vi "Tip tune ZaberAndSR865.vi"(0 "Z axis":T3={"Serial port handle"="", "Axis"="", "Controller #"=0, "Min position"=0.0, "Max position"=0.0, "Min velocity"=0.0, "Max velocity"=0.0, "Firmware"="", "Device ID"=0, "Variable event"=refnum, "Variable ref"=refnum, "Resolution, usteps/step"=0, "Serial port semaphore"=refnum, "Joystick buttons"={"MinDir"=1, "MaxDir"=2, "MedSpeed"=5, "HighSpeed"=6}} {"Joystick buttons"."HighSpeed" min=1 max=25 step=1; "Joystick buttons"."MedSpeed" min=1 max=25 step=1; "Joystick buttons"."MaxDir" min=1 max=25 step=1; "Joystick buttons"."MinDir" min=1 max=25 step=1}, 1 "SR865":T1, 2 "Stop event":refnum<user-event>, 5 "error in":errorcluster) -> (19 "error out":errorcluster)   [LabVIEW 2018]
uses:
  Zaber library/Zaber.ctl
  GenericDataEvent/GenericEvent.ctl
  Zaber library/ZaberVariables.ctl
  SR865/SR865.ctl
  SR865/OutSineReference.ctl
  SR865/OutSineSource.ctl
  SR865/DataChannel.ctl
  <vilib>/Analysis/6fits.llb/Curve Fitting Criteria.ctl
  <vilib>/Analysis/NI_AAL_SigProc.lvlib
  <vilib>/Analysis/NI_AALBase.lvlib
  <vilib>/Analysis/NI_AALPro.lvlib
panel:
  in  "btnReadSignal":bool
  out "Signal":dbl=100000.0 caption="Signal, mV"
  in  "BtnZ-":bool
  in  "BtnZ+":bool
  in  "ZStep":dbl=0.005 caption="Z step, mm" min=0.0 max=25.0 step=0.01 format="%#.4f"
  in  "btnStartPosScanning":bool caption="stop"
  in  "btnCalculateSlope":bool
  in  "btnCalculateSurfaceLevel":bool
  in  "btnCalculateAirLevel":bool
  out "FrequencyStepRb":dbl=100000.0 caption="Frequency"
  out "PhaseRb":dbl=100000.0 caption="Frequency"
  out "AmplitudeRb":dbl=100000.0 caption="Frequency"
  out "DCOffsetRb":dbl=100000.0 caption="DC offset, V"
  out "SlopeError":dbl=8.6 caption="Slope error, V/mm" min=0.0 max=25.0 step=0.01 format="%#.4f"
  out "SurfaceError":dbl=8.6 caption="Surface error, V" min=0.0 max=25.0 step=0.01 format="%#.4f"
  out "AirError":dbl=8.6 caption="Air error, V" min=0.0 max=25.0 step=0.01 format="%#.4f"
  out "Slope":dbl=8.6 caption="Slope, mm/V" min=0.0 max=25.0 step=0.01 format="%#.4f"
  out "SurfaceLevel":dbl=8.6 caption="Surface level, V" min=0.0 max=25.0 step=0.01 format="%#.4f"
  out "AirLevel":dbl=8.6 caption="Air level, V" min=0.0 max=25.0 step=0.01 format="%#.4f"
  out "CurrentStep":i32=61 caption="Z steps"
  out "PltScanningPosition":cluster{dbl[], dbl[]}[](graph) caption="Position scanning"
  out "ZStep":dbl=0.0016666666666666607 caption="Z step, mm" min=0.0 max=25.0 format="%#.4f"
  in  "Frequency":dbl=97044.98 caption="Frequency, Hz" format="%.2p"
  in  "BtnSetZEndPosition":bool
  in  "BtnSetZStartPosition":bool
  in  "ZPoints":i32=61 caption="Z points"
  out "ZEndPosition":dbl=8.6 caption="Z end, mm" min=0.0 max=25.0 format="%#.4f"
  out "ZStartPosition":dbl=8.5 caption="Z start, mm" min=0.0 max=25.0 format="%#.4f"
  out "ZPositionRb":dbl=8.6 caption="Z position" min=0.0 max=25.0 step=0.01 format="%#.4f"
  in  "ZPosition":dbl=8.5 caption="Z position, mm" min=0.0 max=25.0 step=0.01 format="%#.4f"
  out "TblBestFrequencyies":string[][](table)=[["97044.98", "2.85"], ["82864.39", "1.68"], ["21141.21", "1.26"], ["93904.03", "0.82"], ["15778.11", "0.52"]] caption="Best frequencies, Hz"
  in  "TipPlace":u16(ring)=1 caption="Tip place" items=["Air", "Surface"]
  in  "SettingTime":u32=1000 caption="Setting time, ms"
  out "FrequencyRb":dbl=100000.0 caption="Frequency"
  out "CurrentPoint":i32=90
  out "PltScanningFrequence":cluster{dbl[], dbl[]}[](graph)=[{[10000.0, 11000.0, 12000.0, 13000.0, 14000.0, 15000.0, 16000.0, 17000.0, 18000.0, 19000.0, 20000.0, 21000.0, 22000.0, 23000.0, 24000.0, 25000.0, 26000.0, 27000.0, 28000.0, 29000.0, 30000.0, 31000.0, 32000.0, 33000.0, 34000.0, 35000.0, 36000.0, 37000.0, 38000.0, 39000.0, 40000.0, 41000.0, 42000.0, 43000.0, 44000.0, 45000.0, 46000.0, 47000.0, 48000.0, 49000.0, 50000.0, 51000.0, 52000.0, 53000.0, 54000.0, 55000.0, 56000.0, 57000.0, 58000.0, 59000.0, 60000.0, 61000.0, 62000.0, 63000.0, 64000.0, 65000.0, 66000.0, 67000.0, 68000.0, 69000.0, 70000.0, 71000.0, 72000.0, 73000.0, 74000.0, 75000.0, 76000.0, 77000.0, 78000.0, 79000.0, 80000.0, 81000.0, 82000.0, 83000.0, 84000.0, 85000.0, 86000.0, 87000.0, 88000.0, 89000.0, 90000.0, 91000.0, 92000.0, 93000.0, 94000.0, 95000.0, 96000.0, 97000.0, 98000.0, 99000.0, 100000.0], [3.5655190000512516, 3.4374305005139005, 3.4273711461139715, 3.4850248112142093, 3.5761130550998383, 3.556590231281875, 3.5082421792498932, 3.012145327734691, 3.60479334690102, 3.6237170567298436, 3.5213679819034964, 4.863866373270507, 4.004233765623082, 3.958662171251218, 3.638372868429504, 3.6863311988676024, 3.6407628928169347, 3.597268956374069, 3.472475578654757, 3.4138362740831423, 4.023460288827825, 3.8711427099095466, 3.8072787456116726, 3.773067870768127, 3.802872335674139, 3.843425482975206, 3.8131604010931146, 3.710485915669144, 3.68892415072003, 3.7175819077370553, 3.6497045488279003, 3.698426272759254, 3.738228894609222, 3.7572105957332433, 3.841541162636644, 3.552982648310411, 3.6359506328697484, 3.7367182179969376, 3.817937233155462, 3.940743403433729, 4.337961900873752, 3.232249392203631, 3.031809835447508, 3.1009883283630275, 3.1785447948663723, 2.9738534939166783, 3.794967857187948, 3.786370846678634, 3.691365712894553, 3.655859990170908, 3.6562916119155986, 3.5957679438322634, 3.593065477052433, 3.5925726553448727, 3.5922634338806207, 3.590250273321926, 3.597758557035468, 3.5946888897478324, 3.606027010467748, 3.573291409437125, 3.5650938203985896, 3.532467740941366, 3.385655269781037, 3.651862657728945, 3.6418741576807374, 3.5802843235408948, 3.611222575631784, 3.5164236610651676, 4.632535226763082, 3.2424697969441687, 3.272032610844888, 3.3549199729897623, 3.7972193768166784, 5.452081044437504, 2.748058067103696, 2.9130046647694234, 2.9576226283303546, 3.0336329490386387, 3.0499346821806705, 2.9810010016675736, 2.8330872460617447, 2.3801761264752517, 1.3887019949256822, 6.48560906859755, 5.721885978735551, 3.7523307011355125, 2.996072291328326, 5.390088024437564, 5.438011320322094, 4.595058047439225, 4.5440910275334865]}, {[10000.0, 11000.0, 12000.0, 13000.0, 14000.0, 15000.0, 16000.0, 17000.0, 18000.0, 19000.0, 20000.0, 21000.0, 22000.0, 23000.0, 24000.0, 25000.0, 26000.0, 27000.0, 28000.0, 29000.0, 30000.0, 31000.0, 32000.0, 33000.0, 34000.0, 35000.0, 36000.0, 37000.0, 38000.0, 39000.0, 40000.0, 41000.0, 42000.0, 43000.0, 44000.0, 45000.0, 46000.0, 47000.0, 48000.0, 49000.0, 50000.0, 51000.0, 52000.0, 53000.0, 54000.0, 55000.0, 56000.0, 57000.0, 58000.0, 59000.0, 60000.0, 61000.0, 62000.0, 63000.0, 64000.0, 65000.0, 66000.0, 67000.0, 68000.0, 69000.0, 70000.0, 71000.0, 72000.0, 73000.0, 74000.0, 75000.0, 76000.0, 77000.0, 78000.0, 79000.0, 80000.0, 81000.0, 82000.0, 83000.0, 84000.0, 85000.0, 86000.0, 87000.0, 88000.0, 89000.0, 90000.0, 91000.0, 92000.0, 93000.0, 94000.0, 95000.0, 96000.0, 97000.0, 98000.0, 99000.0, 100000.0], [3.6968028657407785, 3.397109339181018, 3.567193952093816, 3.4622519508906793, 3.5945342790368535, 3.5386940424582525, 3.029648511216874, 3.7294031949868516, 3.854496267967221, 3.66608362794549, 3.6337442084525384, 3.622335223134029, 3.520269601833684, 3.625449985669437, 3.5996783070122036, 3.596367060420739, 3.6706800775467205, 3.6178547324397927, 3.494530145248237, 3.4783507835572123, 3.9798696462301795, 3.909521653058709, 3.84636309009401, 3.8283541416529783, 3.8855956102501024, 3.948232372330415, 3.8955390259265563, 3.7044271046719377, 3.6476140823855085, 3.685313344462496, 3.639751480735465, 3.690521795627914, 3.727960158953497, 3.75535848669949, 3.8145229094921054, 3.5935582988975963, 3.6440902453414807, 3.730672290482194, 3.7940627371494946, 3.884890197869988, 4.123519414820418, 5.233578709141258, 2.8898807738384256, 2.709737263826195, 3.650699858167375, 3.6058691787236263, 3.5725795559217843, 3.585563635600408, 3.5978873993164835, 3.6012115301523817, 3.545358407800998, 3.557833559064785, 3.5697611313701043, 3.5699866053317777, 3.5644109564113067, 3.568540350922504, 3.570524521787714, 3.5653418417511418, 3.5472878205078633, 3.566549737959607, 3.5284381997956884, 3.443283156254747, 3.726391503493266, 3.6588555739683373, 3.5487920538102036, 3.744426212291304, 3.774333747133092, 3.7278280955270975, 4.291694487008893, 3.381445353898666, 3.4274420088262834, 3.5326255726860984, 3.8970271568359123, 3.8148611207822927, 4.140697353288415, 3.4812175242568655, 3.7482206201906454, 2.959581027358073, 2.755453572987086, 2.842289778548217, 2.8230407994627473, 2.5397852639697267, 1.7720535165304037, 6.311279502338936, 4.911483553972613, 3.8801745664846505, 3.1735908186482717, 2.5479667164400683, 5.117117280660982, 5.956381695510879, 6.236143926446963]}, {[10000.0, 11000.0, 12000.0, 13000.0, 14000.0, 15000.0, 16000.0, 17000.0, 18000.0, 19000.0, 20000.0, 21000.0, 22000.0, 23000.0, 24000.0, 25000.0, 26000.0, 27000.0, 28000.0, 29000.0, 30000.0, 31000.0, 32000.0, 33000.0, 34000.0, 35000.0, 36000.0, 37000.0, 38000.0, 39000.0, 40000.0, 41000.0, 42000.0, 43000.0, 44000.0, 45000.0, 46000.0, 47000.0, 48000.0, 49000.0, 50000.0, 51000.0, 52000.0, 53000.0, 54000.0, 55000.0, 56000.0, 57000.0, 58000.0, 59000.0, 60000.0, 61000.0, 62000.0, 63000.0, 64000.0, 65000.0, 66000.0, 67000.0, 68000.0, 69000.0, 70000.0, 71000.0, 72000.0, 73000.0, 74000.0, 75000.0, 76000.0, 77000.0, 78000.0, 79000.0, 80000.0, 81000.0, 82000.0, 83000.0, 84000.0, 85000.0, 86000.0, 87000.0, 88000.0, 89000.0, 90000.0, 91000.0, 92000.0, 93000.0, 94000.0, 95000.0, 96000.0, 97000.0, 98000.0, 99000.0, 100000.0], [-0.131283865689527, 0.04032116133288266, -0.1398228059798443, 0.022772860323529986, -0.018421223937015174, 0.017896188823622428, 0.47859366803301917, -0.7172578672521608, -0.24970292106620118, -0.04236657121564624, -0.112376226549042, 1.2415311501364776, 0.4839641637893983, 0.3332121855817811, 0.03869456141730021, 0.08996413844686346, -0.029917184729785884, -0.02058577606572376, -0.02205456659347993, -0.06451450947407, 0.043590642597645335, -0.03837894314916257, -0.03908434448233722, -0.05528627088485116, -0.0827232745759634, -0.10480688935520899, -0.08237862483344172, 0.0060588109972061766, 0.04131006833452133, 0.03226856327455918, 0.009953068092435124, 0.007904477131339682, 0.01026873565572517, 0.0018521090337535462, 0.02701825314453865, -0.04057565058718504, -0.008139612471732338, 0.006045927514743532, 0.023874496005967583, 0.05585320556374107, 0.2144424860533345, -2.0013293169376274, 0.14192906160908247, 0.39125106453683234, -0.47215506330100254, -0.632015684806948, 0.2223883012661636, 0.2008072110782262, 0.09347831357806946, 0.05464846001852619, 0.1109332041146005, 0.037934384767478235, 0.02330434568232853, 0.022586050013094994, 0.027852477469314074, 0.021709922399422155, 0.02723403524775403, 0.029347047996690634, 0.05873918995988481, 0.006741671477517919, 0.03665562060290117, 0.08918458468661905, -0.3407362337122293, -0.006992916239392244, 0.09308210387053384, -0.16414188875040914, -0.16311117150130805, -0.2114044344619299, 0.3408407397541886, -0.13897555695449748, -0.15540939798139553, -0.17770559969633615, -0.09980778001923385, 1.6372199236552114, -1.392639286184719, -0.568212859487442, -0.7905979918602908, 0.07405192168056551, 0.2944811091935846, 0.13871122311935657, 0.010046446598997338, -0.15960913749447503, -0.3833515216047214, 0.1743295662586144, 0.8104024247629376, -0.12784386534913805, -0.17751852731994555, 2.842121307997496, 0.32089403966111174, -1.3613236480716537, -1.6920528989134764]}] caption="Frequence scanning"
  in  "btnStartFreqScanning":bool caption="stop"
  out "FrequencyPoints":i32=91 caption="Frequency points"
  in  "FrequencyStep":dbl=1000.0 caption="Frequency step, Hz"
  in  "EndFrequency":dbl=100000.0 caption="End frequency, Hz" format="%.2p"
  in  "Phase":dbl format="%.3f"
  in  "StartFrequency":dbl=10000.0 caption="Start frequency, Hz" format="%.2p"
  in  "Amplitude":dbl=0.5 caption="Amplitude p-p, V" min=0.0 max=10.0 format="%.3f"
  # "RS865 parameters"
  # "Z stage parameters"
  # "Scanning parameters"
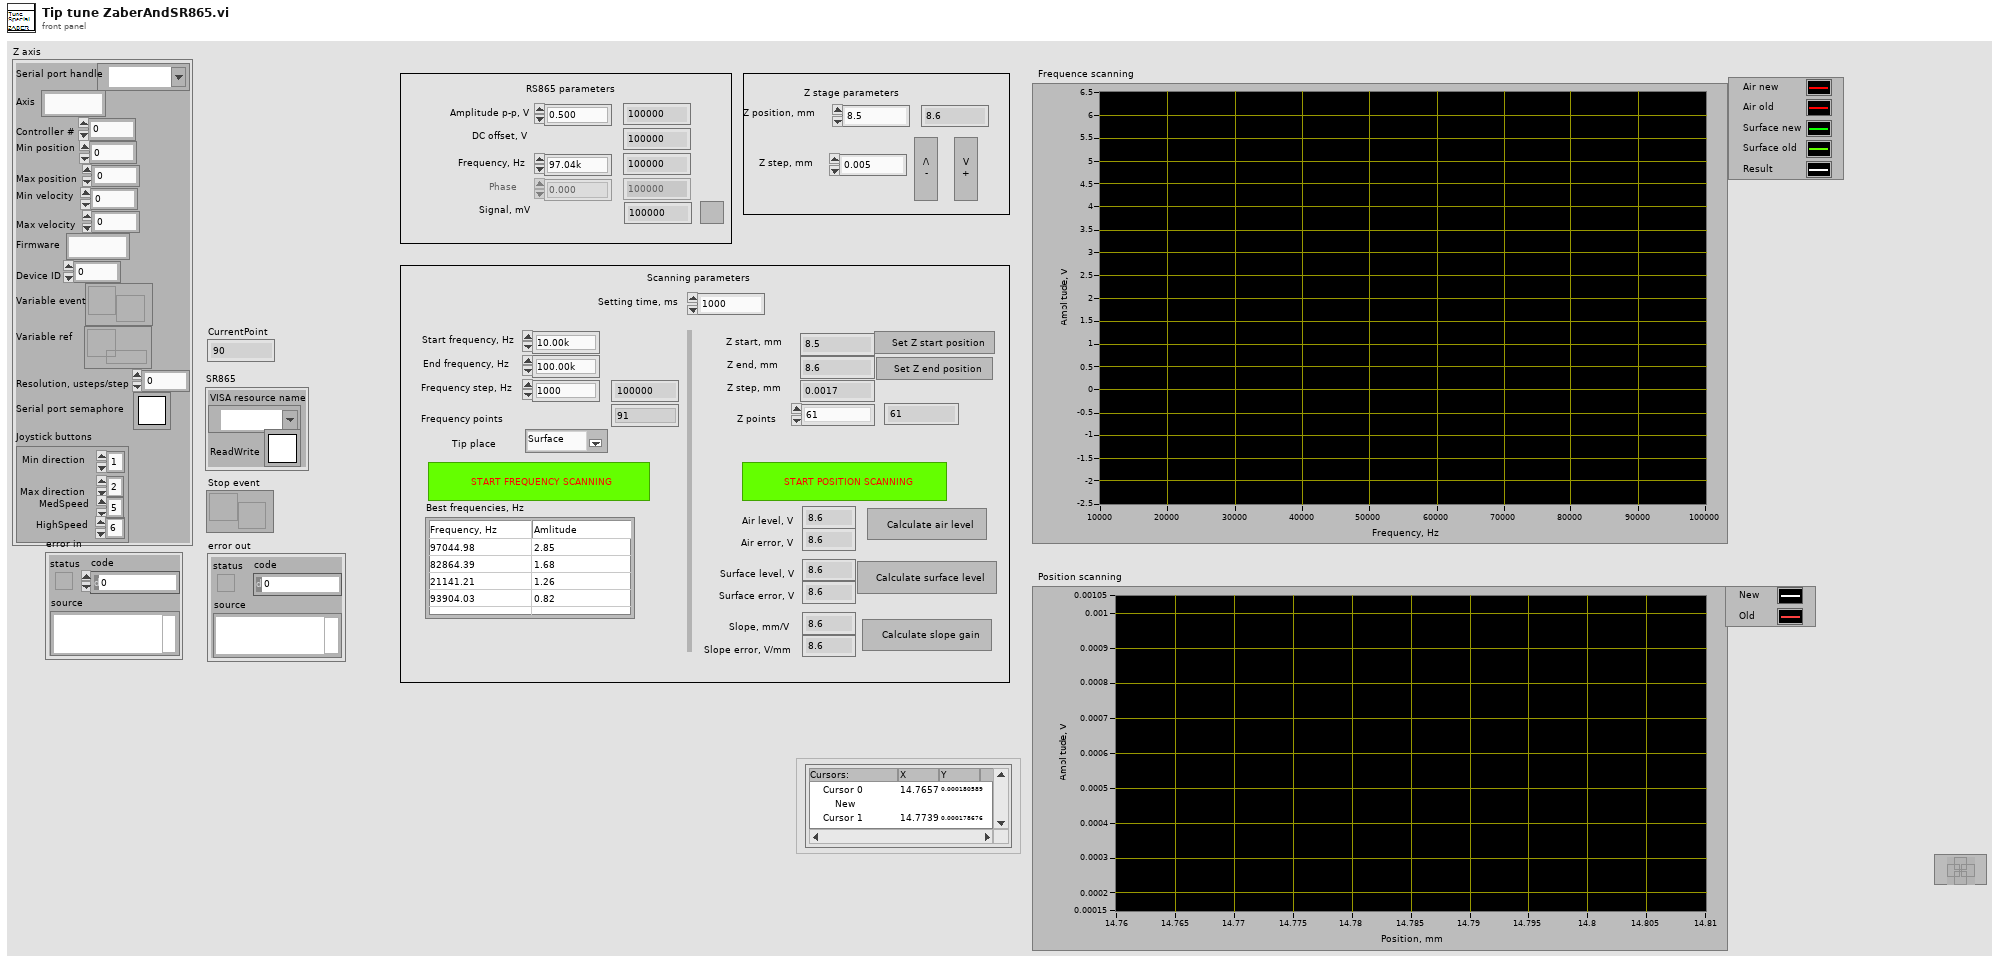
[diagram p1: front panel]
types:
  T1 = typedef "SR865.ctl" = cluster{"VISA resource name":refnum<visa-resource-name>, "ReadWrite":T2}
  T2 = typedef "Semaphore RefNum" = refnum<k1>
  T3 = typedef "Zaber.ctl" = cluster{"Serial port handle":refnum<visa-resource-name>, "Axis":string, "Controller #":u8, "Min position":dbl, "Max position":dbl, "Min velocity":dbl, "Max velocity":dbl, "Firmware":string, "Device ID":i32, "Variable event":T4, "Variable ref":refnum<data-value>, "Resolution, usteps/step":i32, "Serial port semaphore":T2, "Joystick buttons":cluster{"MinDir":i32, "MaxDir":i32, "MedSpeed":i32, "HighSpeed":i32}}
  T4 = typedef "GenericEvent.ctl" = refnum<user-event>
  T5 = typedef "DataChannel.ctl" = u16
  T6 = typedef "OutSineSource.ctl" = u16
  T7 = typedef "OutSineReference.ctl" = u16
  T8 = typedef "LVCursorListTypeDef.ctl" = cluster{"Name":string, "Color":u32, "Style":u8, "Point Style":u8, "Name Visible":bool, "Allow Drag":bool, "Cursor Mode":u32, "Plot":i32, "Index":i32, "Position":cluster{"X":dbl, "Y":dbl}, "X Scale":u32, "Y Scale":u32, "Watch Plots":i32[], "Watch All Plots":bool, "Plot Area":i32, "Label Offset":cluster{"X":dbl, "Y":dbl}}[]
  T9 = cluster{"Name":string, "Color":u32, "Style":u8, "Point Style":u8, "Name Visible":bool, "Allow Drag":bool, "Cursor Mode":u32, "Plot":i32, "Index":i32, "Position":cluster{"X":dbl, "Y":dbl}, "X Scale":u32, "Y Scale":u32, "Watch Plots":i32[], "Watch All Plots":bool, "Plot Area":i32, "Label Offset":cluster{"X":dbl, "Y":dbl}}
  T10 = typedef "NI_AALPro.lvlib/Curve Fitting Criteria.ctl" = u16
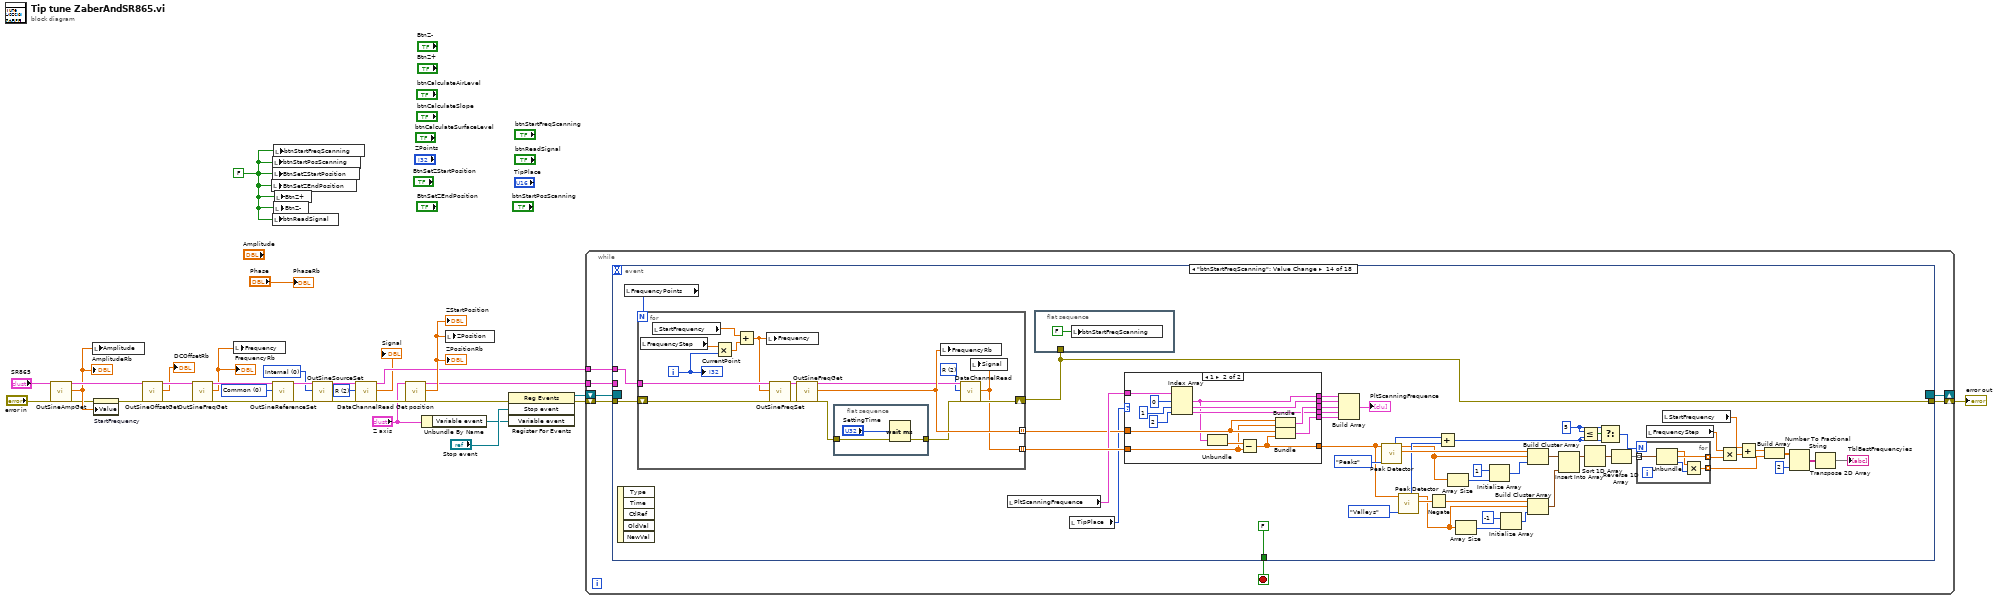
[diagram p0: block diagram]
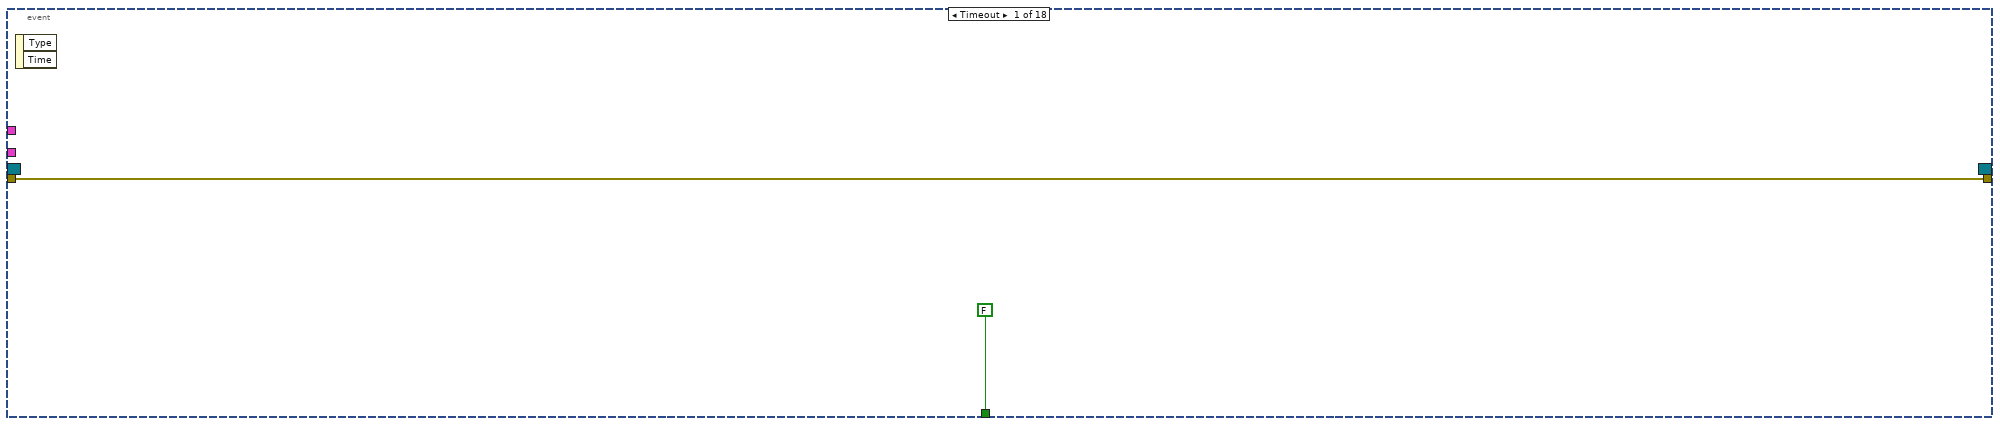
[diagram p2: hidden frame]
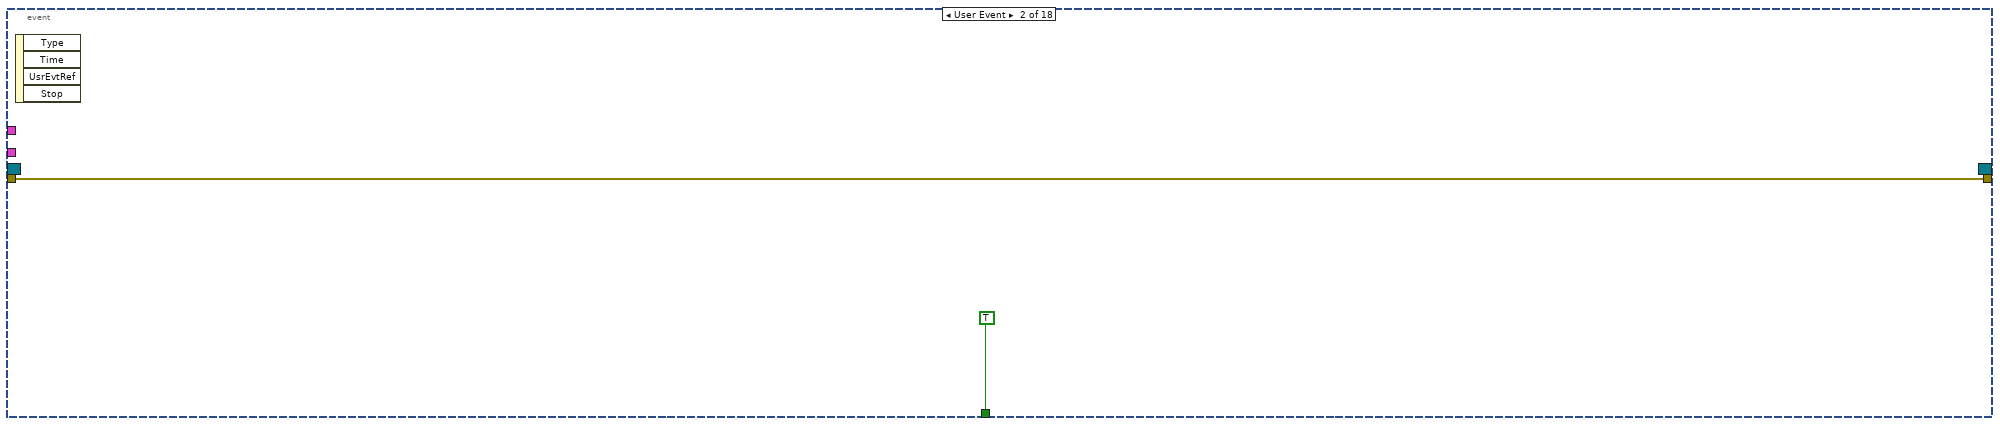
[diagram p3: hidden frame]
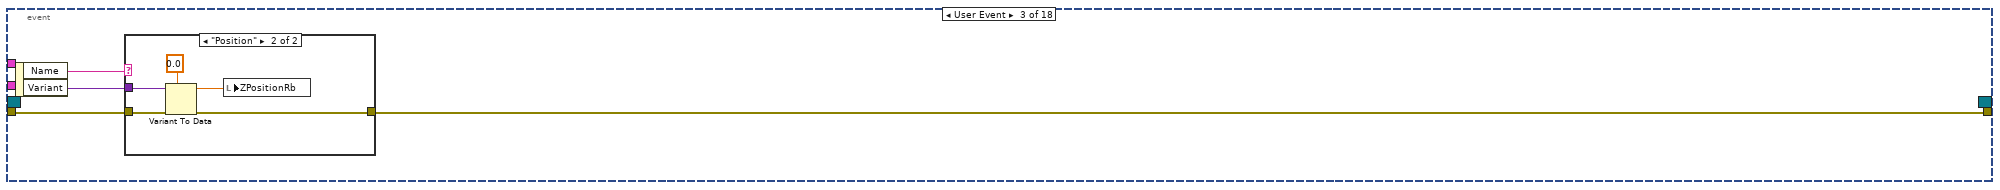
[diagram p4: hidden frame]
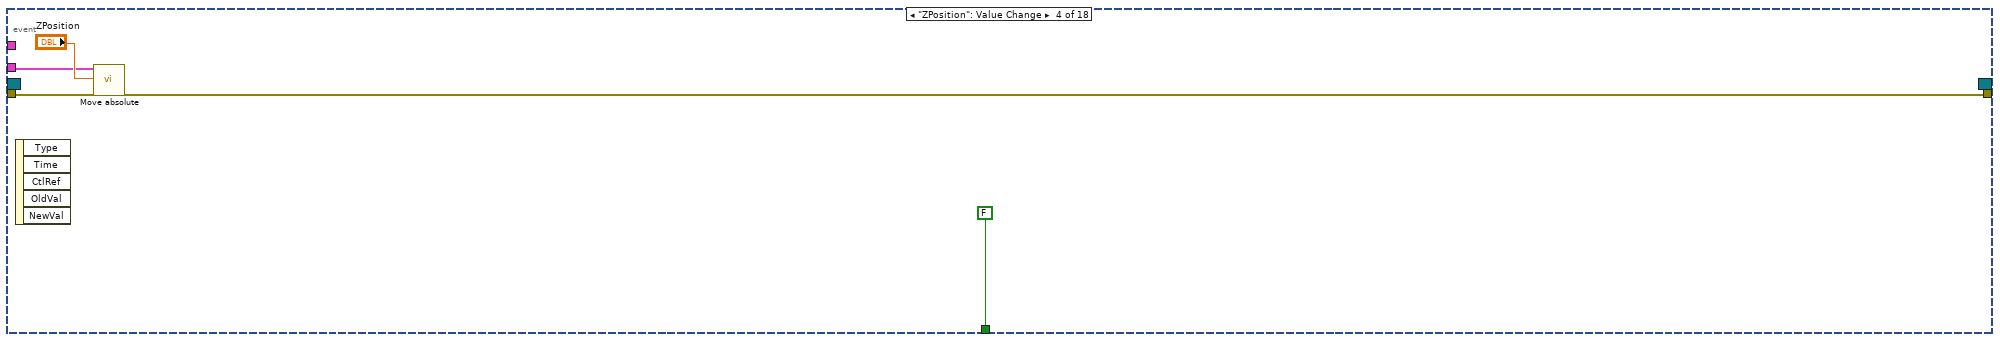
[diagram p6: hidden frame]
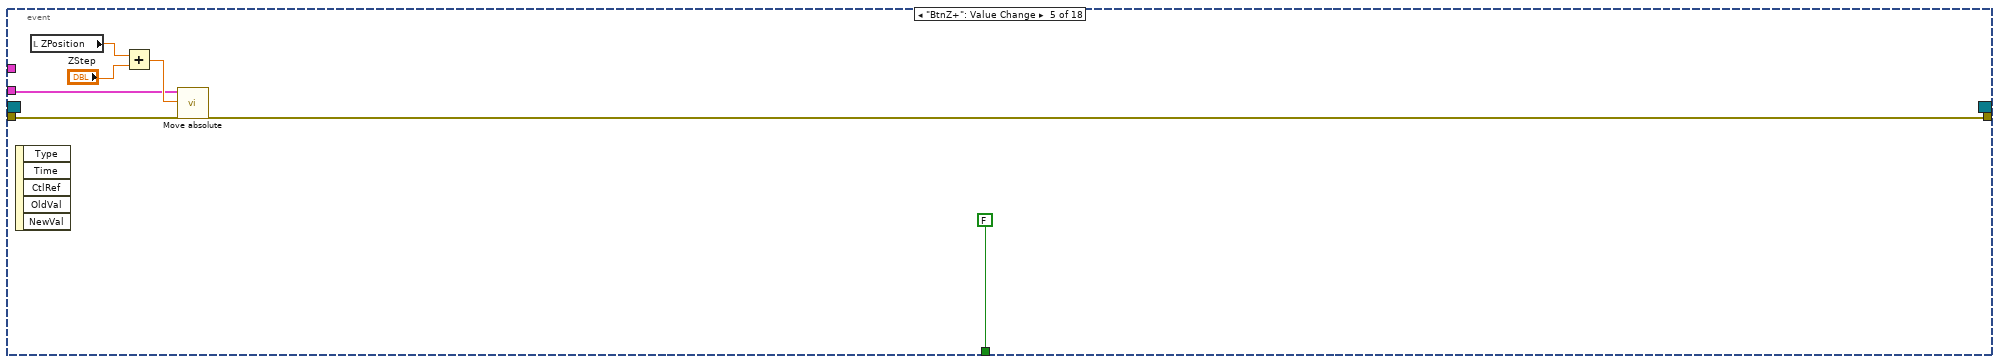
[diagram p7: hidden frame]
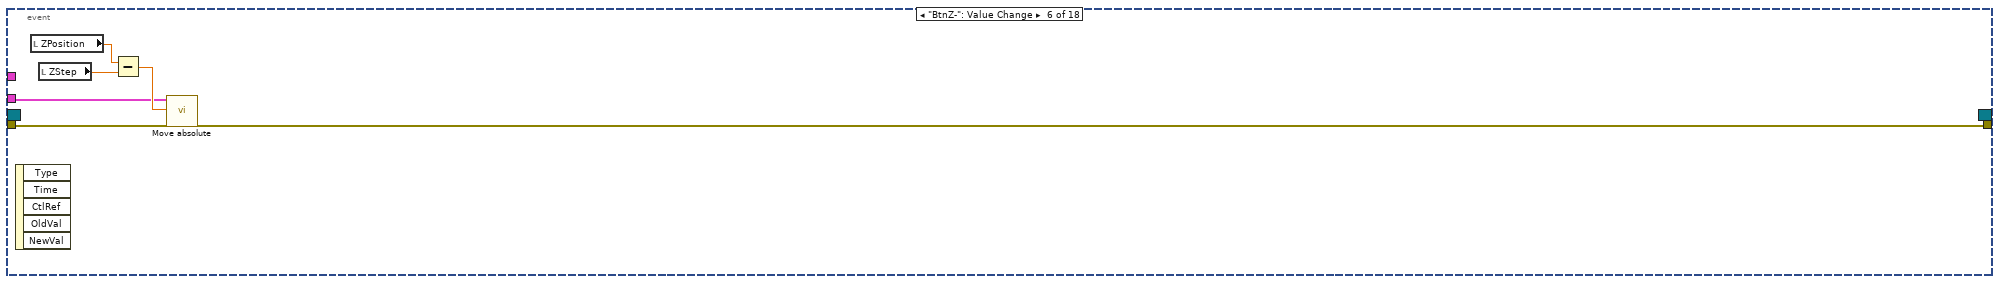
[diagram p8: hidden frame]
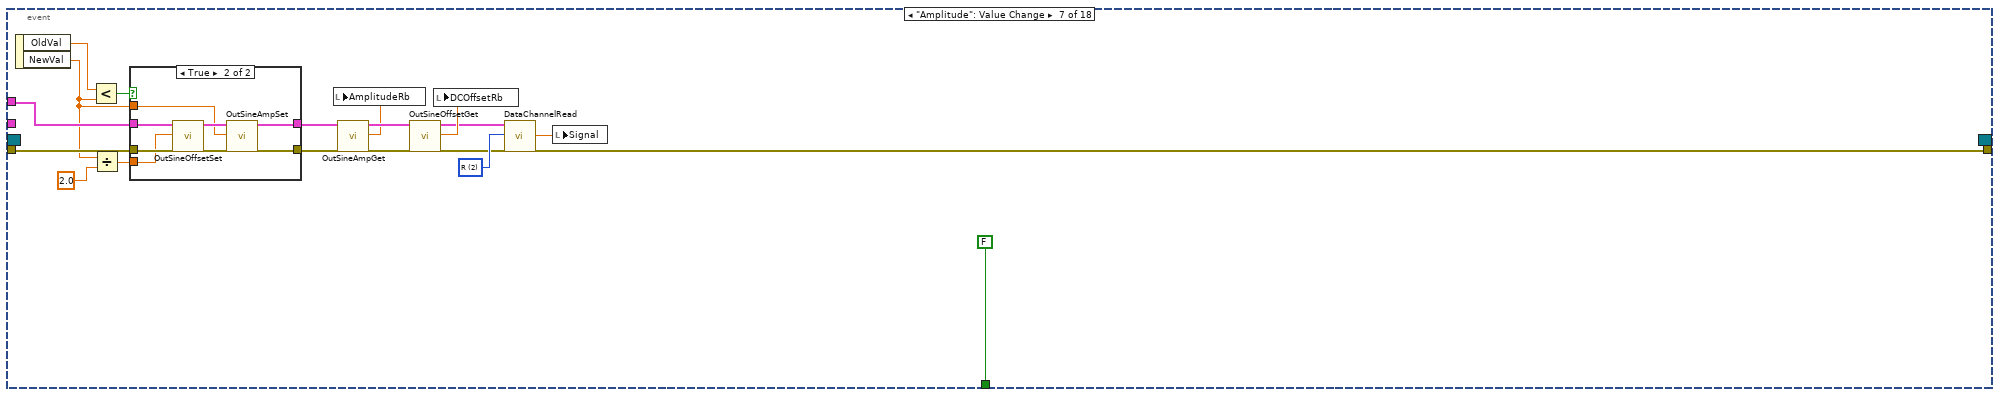
[diagram p9: hidden frame]
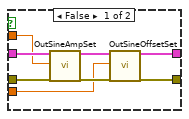
[diagram p10: hidden frame]
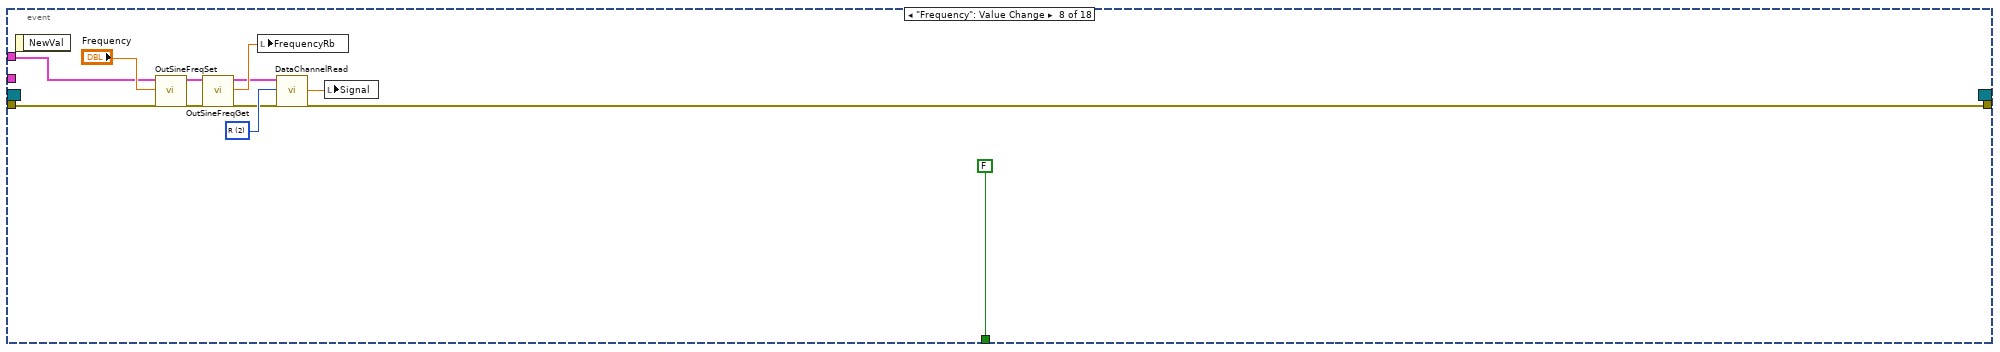
[diagram p11: hidden frame]
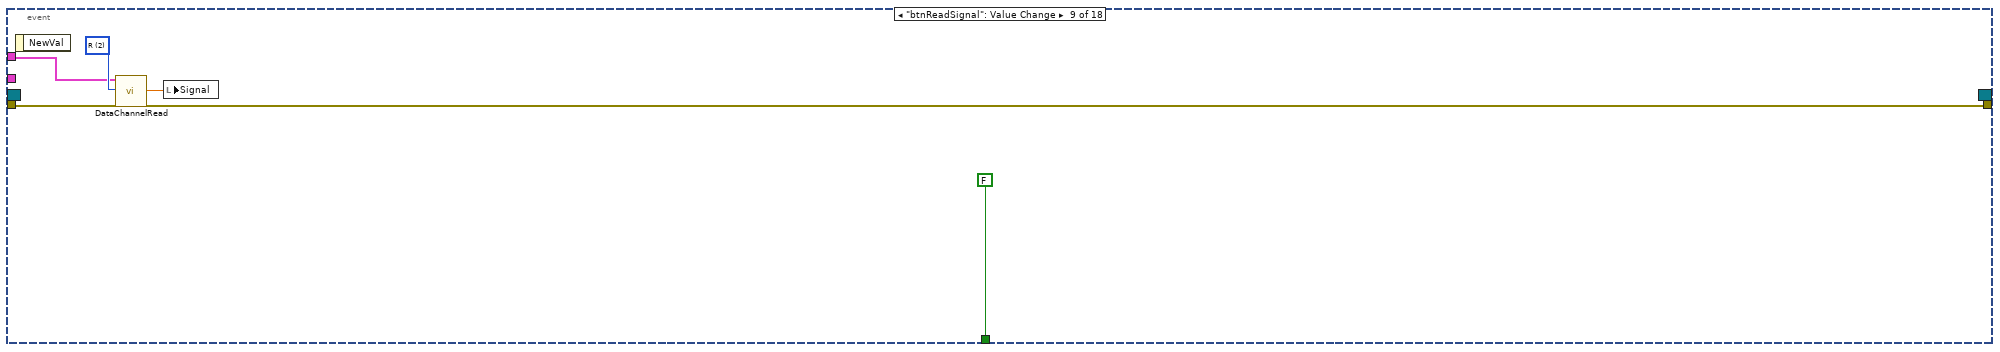
[diagram p12: hidden frame]
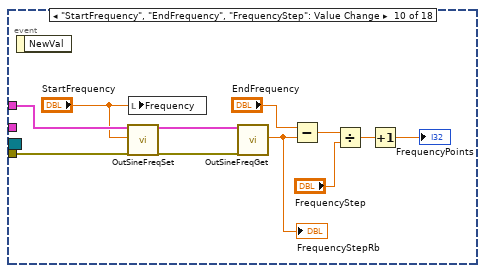
[diagram p13: hidden frame]
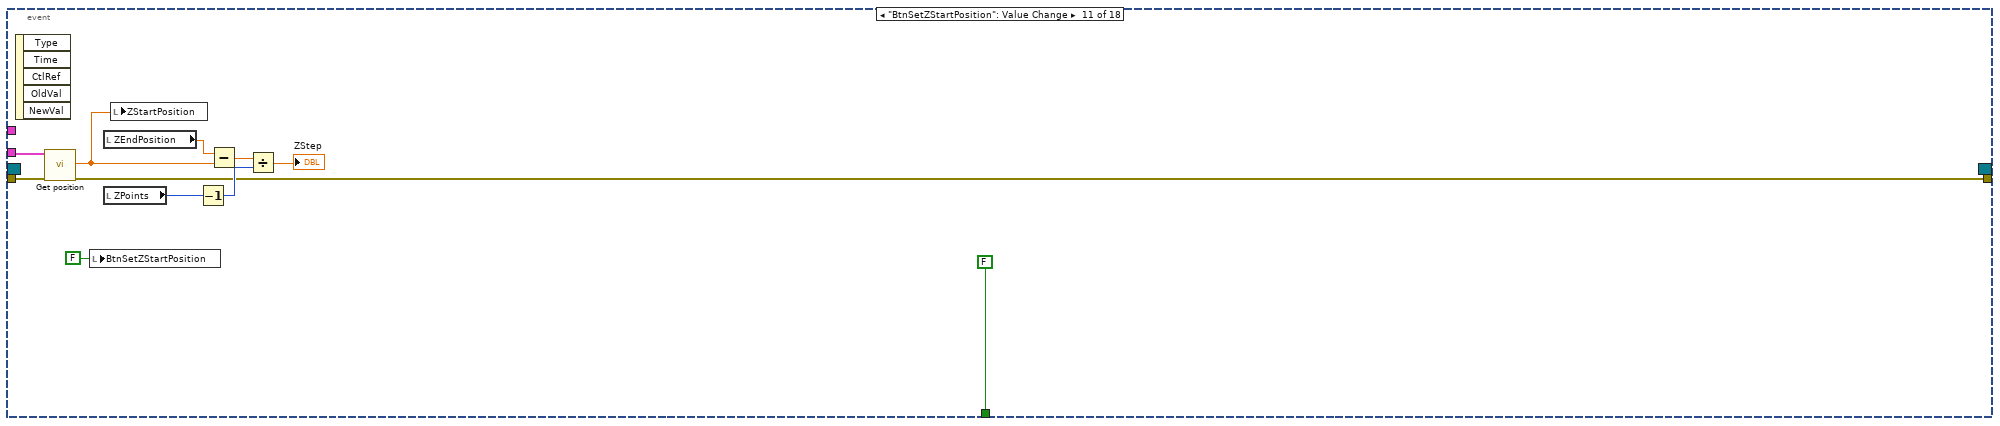
[diagram p14: hidden frame]
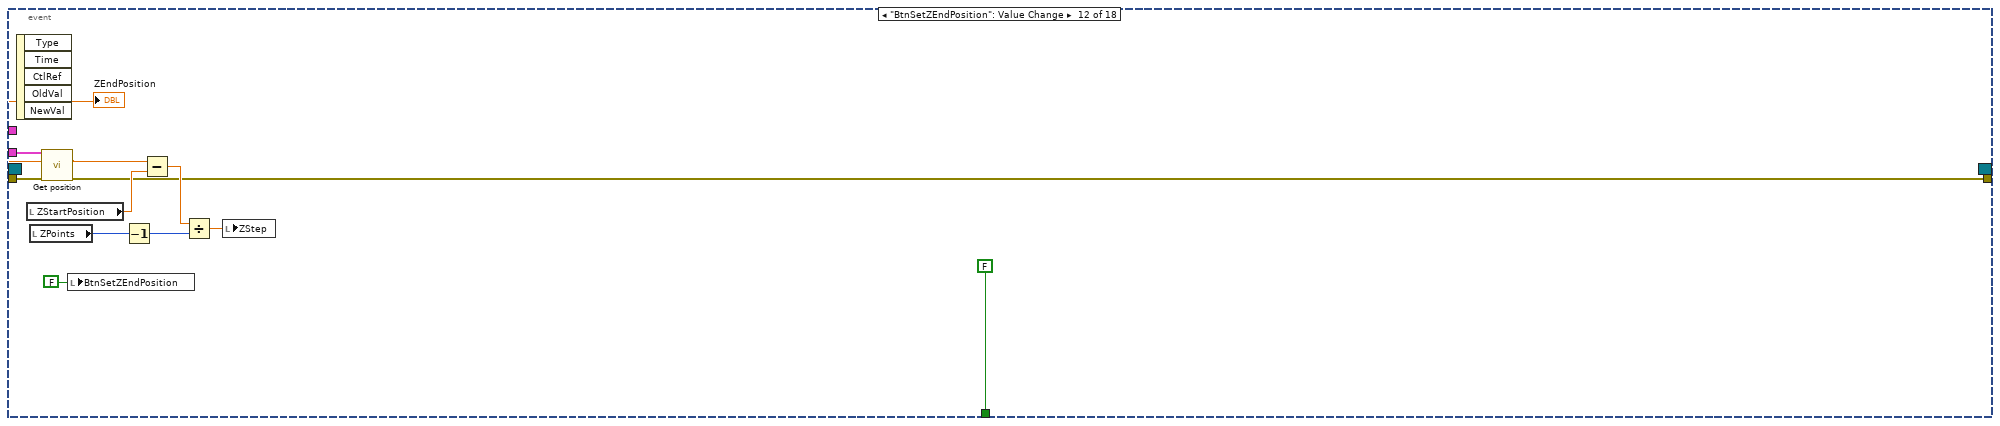
[diagram p15: hidden frame]
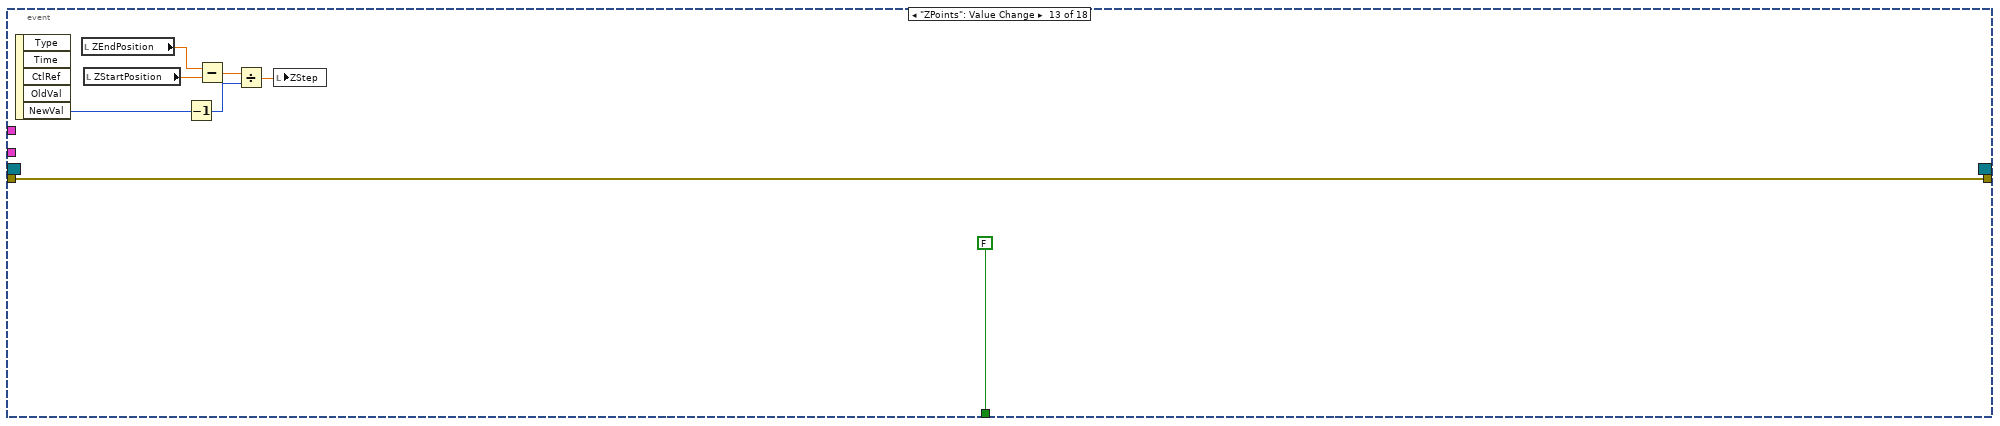
[diagram p16: hidden frame]
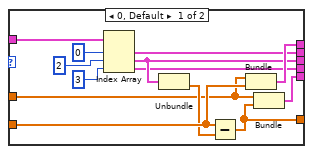
[diagram p17: hidden frame]
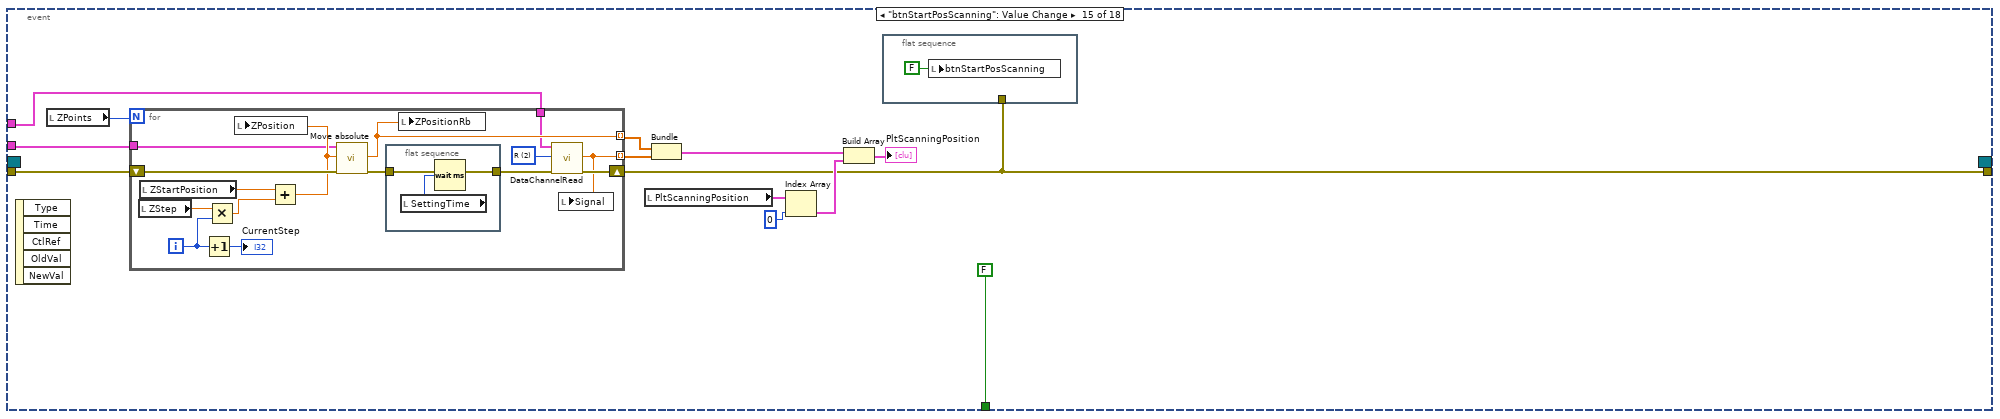
[diagram p18: hidden frame]
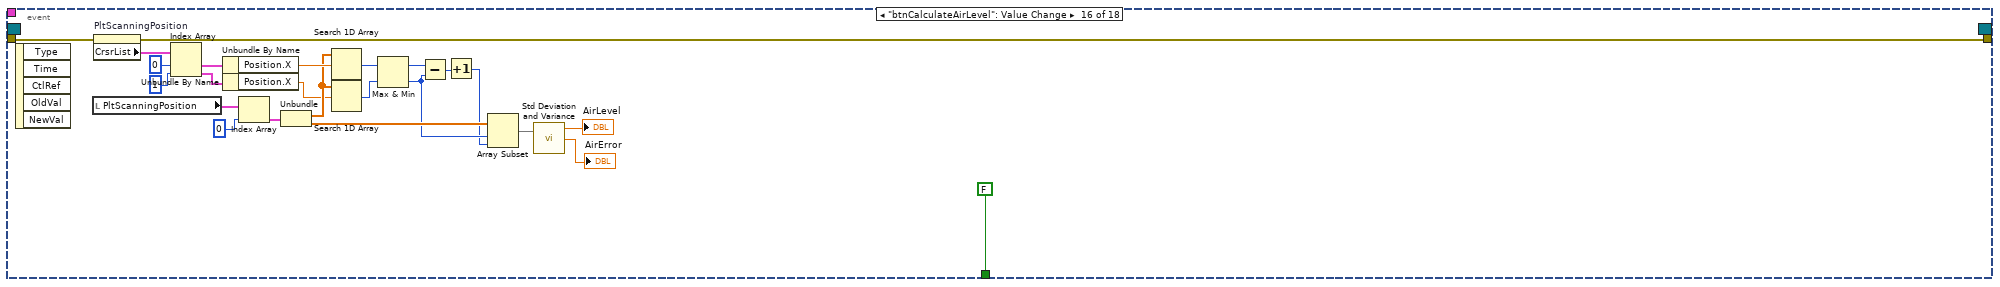
[diagram p19: hidden frame]
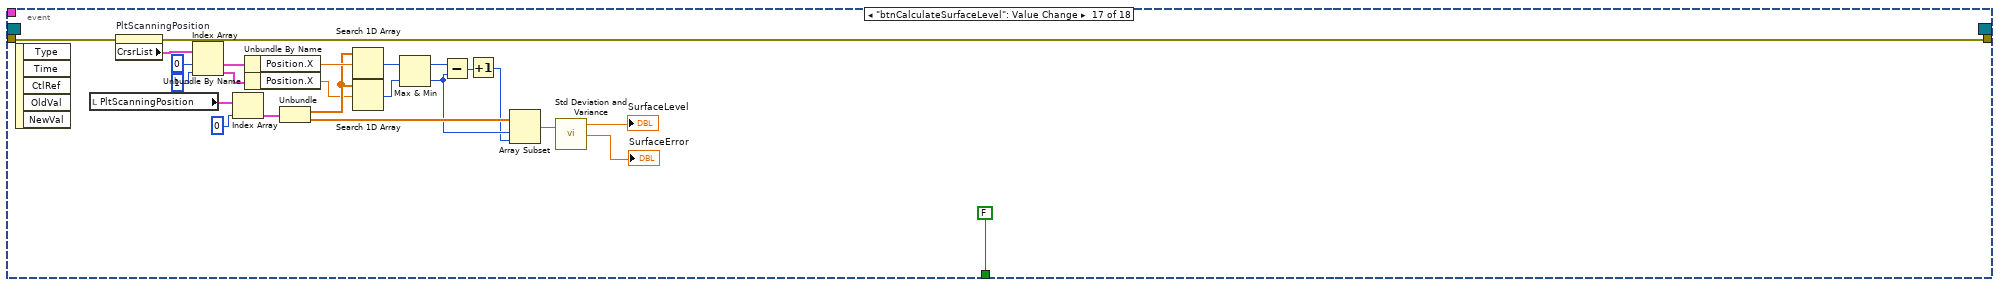
[diagram p20: hidden frame]
diagram:
  w12 = T5 2 items=["X", "Y", "R", "Theta", "IN1", "IN2", "IN3", "IN4", "OUT1", "OUT2", "XNoise", "YNoise", "Phase", "SineOut", "DCLevel", "IntRefFreq", "ExtRefFreq"] ("DataChannel")
  w20 = T6 0 items=["Internal", "External", "Dual", "Chop"] ("OutSineSource")
  w23 = T7 0 items=["Common", "Difference"] ("OutSineRef")
  w7 = FALSE ("btnStartStop")
  n1 = call "OutSineAmpGet.vi"("SR865 in"="SR865", "error in"="error in") -> ("SR865 out"=w30:T1, "Amplitude"=w17:dbl, "error out"=w16:errorcluster)  [unwired: 15 in]
  "AmplitudeRb" <- w17
  n2 = local write "Amplitude"(w17) -> ()
  n3 = property on="StartFrequency" class="DigNum (strict)"(error in=w16, "Value"=w17) -> (error out=w15:errorcluster)  [unwired: 1 in, 1 out]
  n4 = call "OutSineOffsetGet.vi"("SR865 in"=w30, "error in"=w15) -> ("SR865 out"=w29:T1, "Offset"=→"DCOffsetRb":dbl, "error out"=w28:errorcluster)  [unwired: 15 in]
  n5 = call "OutSineFreqGet.vi"("SR865 in"=w29, "error in"=w28) -> ("SR865 out"=w24:T1, "Frequency"=w13:dbl, "error out"=w25:errorcluster)  [unwired: 15 in]
  "FrequencyRb" <- w13
  n6 = local write "Frequency"(w13) -> ()
  n7 = local write "BtnSetZEndPosition"(w7) -> ()
  n8 = local write "btnStartPosScanning"(w7) -> ()
  n9 = local write "BtnSetZStartPosition"(w7) -> ()
  n10 = local write "btnReadSignal"(w7) -> ()
  n11 = call "OutSineReferenceSet.vi"("SR865 in"=w24, "OutSineRef"=w23, "error in"=w25) -> ("SR865 out"=w21:T1, "error out"=w22:errorcluster)  [unwired: 15 in]
  n12 = local write "btnStartFreqScanning"(w7) -> ()
  n13 = local write "BtnZ-"(w7) -> ()
  n14 = local write "BtnZ+"(w7) -> ()
  n15 = call "OutSineSourceSet.vi"("SR865 in"=w21, "OutSineSource"=w20, "error in"=w22) -> ("SR865 out"=w10:T1, "error out"=w11:errorcluster)  [unwired: 15 in]
  n16 = call "DataChannelRead.vi"("SR865 in"=w10, "DataChannel"=w12, "error in"=w11) -> ("SR865 out"=w9:T1, "Signal"=→"Signal":dbl, "error out"=w5:errorcluster)  [unwired: 14 in]
  n17 = call "Get position.vi"("Zaber"="Z axis", "error in"=w5) -> ("Zaber out"=w3:T3, "PositionRb"=w14:dbl, "error out"=w4:errorcluster)  [unwired: 13 in, 2 out]
  "ZPositionRb" <- w14
  "ZStartPosition" <- w14
  n18 = Unbundle By Name("Z axis") -> ("Variable event"=w1:T4)
  n19 = local write "ZPosition"(w14) -> ()
  n20 = register-events(error in=w4, "Stop event", w1) -> (reference out=w32:refnum<event-registration>, error out=w18:errorcluster)  [unwired: 1 in]
  n21 = while {
    tunnel: w9 -> [w40]
    tunnel: w3 -> [w37]
    shift-right: [w38] -> w6
    shift-left: w18 -> [w39]
    shift-right: [w34] -> _
    shift-left: w32 -> [w36]
    stop <- w35 stop-if-true
    n22 = event shown="[13] \"btnStartFreqScanning\": Value Change" {
      selector: w36 -> [_ _ _ _ _ _ _ _ _ _ _ _ _ _ _ _ _ _]
      dyn-events: [_ _ _ _ _ _ _ _ _ _ _ _ _ _ _ _ _ _] -> w34
      timeout: _ -> [_ _ _ _ _ _ _ _ _ _ _ _ _ _ _ _ _ _]
      tunnel: w40 -> [_ _ _ _ _ _ w89 w118 w123 w134 _ _ _ w216 w270 _ _ _]
      tunnel: w39 -> [w42 w43 w48 w58 w66 w70 w90 w117 w124 w133 w141 w152 w159 w215 w271 w303 w327 w351]
      tunnel: [w42 w43 w47 w57 w62 w69 w74 w109 w121 _ w140 w151 w159 w213 w267 w302 w326 w350] -> w38
      tunnel: w37 -> [_ _ _ w55 w60 w67 _ _ _ _ w137 w148 _ _ w269 _ _ _]
      tunnel: [FALSE TRUE _ FALSE FALSE _ FALSE FALSE FALSE _ FALSE FALSE FALSE FALSE FALSE FALSE FALSE FALSE] -> w35
      event Timeout {
        n23 = event-data() -> ()  [unwired: 1 in, 2 out]
      }
      event User Event {
        n24 = event-data() -> ()  [unwired: 1 in, 4 out]
      }
      event User Event {
        n25 = event-data() -> ("Name"=w45:string, "Variant"=w46:variant)  [unwired: 1 in]
        n26 = case shown="\"Position\"" w45 {
          tunnel: w48 -> [w49 w52]
          tunnel: [w49 w51] -> w47
          tunnel: w46 -> [_ w50]
          frame Default {
          }
          frame "Position" {
            n27 = Variant To Data(error in=w52, type=0.0, Variant=w50) -> (data=w53:dbl, error out=w51:errorcluster)
            n28 = local write "ZPositionRb"(w53) -> ()
          }
        }
      }
      event "ZPosition": Value Change {
        n29 = event-data() -> ()  [unwired: 1 in, 5 out]
        n30 = call "Move absolute.vi"("Zaber"=w55, "Position, mm"="ZPosition", "error in"=w58) -> ("error out"=w57:errorcluster)  [unwired: 13 in, 3 out]
      }
      event "BtnZ+": Value Change {
        n31 = event-data() -> ()  [unwired: 1 in, 5 out]
        n32 = local read "ZPosition"() -> (w65:dbl)
        n33 = Add(x=w65, y="ZStep") -> (x+y=w63:dbl)
        n34 = call "Move absolute.vi"("Zaber"=w60, "Position, mm"=w63, "error in"=w66) -> ("error out"=w62:errorcluster)  [unwired: 13 in, 3 out]
      }
      event "BtnZ-": Value Change {
        n35 = event-data() -> ()  [unwired: 1 in, 5 out]
        n36 = local read "ZPosition"() -> (w72:dbl)
        n37 = local read "ZStep"() -> (w68:dbl)
        n38 = Subtract(x=w72, y=w68) -> (x-y=w71:dbl)
        n39 = call "Move absolute.vi"("Zaber"=w67, "Position, mm"=w71, "error in"=w70) -> ("error out"=w69:errorcluster)  [unwired: 13 in, 3 out]
      }
      event "Amplitude": Value Change {
        w77 = T5 2 items=["X", "Y", "R", "Theta", "IN1", "IN2", "IN3", "IN4", "OUT1", "OUT2", "XNoise", "YNoise", "Phase", "SineOut", "DCLevel", "IntRefFreq", "ExtRefFreq"] ("DataChannel")
        n40 = event-data() -> ("OldVal"=w87:dbl, "NewVal"=w78:dbl)  [unwired: 1 in]
        n41 = Less?(x=w87, y=w78) -> (x < y?=w88:bool)
        n42 = Divide(x=w78, y=2.0) -> (x/y=w79:dbl)
        n43 = case shown="True" w88 {
          tunnel: w90 -> [w99 w107]
          tunnel: [w97 w105] -> w85
          tunnel: w89 -> [w96 w104]
          tunnel: [w94 w102] -> w83
          tunnel: w78 -> [w93 w101]
          tunnel: w79 -> [w92 w100]
          frame False {
            n44 = call "OutSineAmpSet.vi"("SR865 in"=w96, "Amplitude"=w93, "error in"=w99) -> ("SR865 out"=w95:T1, "error out"=w98:errorcluster)  [unwired: 15 in]
            n45 = call "OutSineOffsetSet.vi"("SR865 in"=w95, "Amplitude"=w92, "error in"=w98) -> ("SR865 out"=w94:T1, "error out"=w97:errorcluster)  [unwired: 15 in]
          }
          frame True {
            n46 = call "OutSineOffsetSet.vi"("SR865 in"=w104, "Amplitude"=w100, "error in"=w107) -> ("SR865 out"=w103:T1, "error out"=w106:errorcluster)  [unwired: 15 in]
            n47 = call "OutSineAmpSet.vi"("SR865 in"=w103, "Amplitude"=w101, "error in"=w106) -> ("SR865 out"=w102:T1, "error out"=w105:errorcluster)  [unwired: 15 in]
          }
        }
        n48 = call "OutSineAmpGet.vi"("SR865 in"=w83, "error in"=w85) -> ("SR865 out"=w84:T1, "Amplitude"=w81:dbl, "error out"=w86:errorcluster)  [unwired: 15 in]
        n49 = local write "AmplitudeRb"(w81) -> ()
        n50 = call "OutSineOffsetGet.vi"("SR865 in"=w84, "error in"=w86) -> ("SR865 out"=w73:T1, "Offset"=w82:dbl, "error out"=w75:errorcluster)  [unwired: 15 in]
        n51 = local write "DCOffsetRb"(w82) -> ()
        n52 = call "DataChannelRead.vi"("SR865 in"=w73, "DataChannel"=w77, "error in"=w75) -> ("Signal"=w76:dbl, "error out"=w74:errorcluster)  [unwired: 14 in, 1 out]
        n53 = local write "Signal"(w76) -> ()
      }
      event "Frequency": Value Change {
        w112 = T5 2 items=["X", "Y", "R", "Theta", "IN1", "IN2", "IN3", "IN4", "OUT1", "OUT2", "XNoise", "YNoise", "Phase", "SineOut", "DCLevel", "IntRefFreq", "ExtRefFreq"] ("DataChannel")
        n54 = event-data() -> ()  [unwired: 1 in, 1 out]
        n55 = call "OutSineFreqSet.vi"("SR865 in"=w118, "Frequency"="Frequency", "error in"=w117) -> ("SR865 out"=w115:T1, "error out"=w116:errorcluster)  [unwired: 15 in]
        n56 = call "OutSineFreqGet.vi"("SR865 in"=w115, "error in"=w116) -> ("SR865 out"=w108:T1, "Frequency"=w114:dbl, "error out"=w110:errorcluster)  [unwired: 15 in]
        n57 = local write "FrequencyRb"(w114) -> ()
        n58 = call "DataChannelRead.vi"("SR865 in"=w108, "DataChannel"=w112, "error in"=w110) -> ("Signal"=w111:dbl, "error out"=w109:errorcluster)  [unwired: 14 in, 1 out]
        n59 = local write "Signal"(w111) -> ()
      }
      event "btnReadSignal": Value Change {
        w125 = T5 2 items=["X", "Y", "R", "Theta", "IN1", "IN2", "IN3", "IN4", "OUT1", "OUT2", "XNoise", "YNoise", "Phase", "SineOut", "DCLevel", "IntRefFreq", "ExtRefFreq"] ("DataChannel")
        n60 = event-data() -> ()  [unwired: 1 in, 1 out]
        n61 = call "DataChannelRead.vi"("SR865 in"=w123, "DataChannel"=w125, "error in"=w124) -> ("Signal"=w122:dbl, "error out"=w121:errorcluster)  [unwired: 14 in, 1 out]
        n62 = local write "Signal"(w122) -> ()
      }
      event "StartFrequency", "EndFrequency", "FrequencyStep": Value Change {
        n63 = event-data() -> ()  [unwired: 1 in, 1 out]
        n64 = call "OutSineFreqSet.vi"("SR865 in"=w134, "Frequency"="StartFrequency", "error in"=w133) -> ("SR865 out"=w135:T1, "error out"=w136:errorcluster)  [unwired: 15 in]
        n65 = local write "Frequency"("StartFrequency") -> ()
        n66 = call "OutSineFreqGet.vi"("SR865 in"=w135, "error in"=w136) -> ("Frequency"=w126:dbl)  [unwired: 15 in, 2 out]
        "FrequencyStepRb" <- w126
        n67 = Subtract(x="EndFrequency", y=w126) -> (x-y=w131:dbl)
        n68 = Divide(x=w131, y="FrequencyStep") -> (x/y=w129:dbl)
        n69 = Increment(x=w129) -> (x+1=→"FrequencyPoints":dbl)
      }
      event "BtnSetZStartPosition": Value Change {
        n70 = event-data() -> ()  [unwired: 1 in, 5 out]
        n71 = call "Get position.vi"("Zaber"=w137, "error in"=w141) -> ("PositionRb"=w138:dbl, "error out"=w140:errorcluster)  [unwired: 13 in, 3 out]
        n72 = local write "BtnSetZStartPosition"(FALSE ("BtnSetZStartPosition")) -> ()
        n73 = local read "ZEndPosition"() -> (w143:dbl)
        n74 = local read "ZPoints"() -> (w145:i32)
        n75 = local write "ZStartPosition"(w138) -> ()
        n76 = Decrement(x=w145) -> (x-1=w144:i32)
        n77 = Subtract(x=w143, y=w138) -> (x-y=w146:dbl)
        n78 = Divide(x=w146, y=w144) -> (x/y=→"ZStep":dbl)
      }
      event "BtnSetZEndPosition": Value Change {
        n79 = event-data() -> ()  [unwired: 1 in, 5 out]
        n80 = local read "ZStartPosition"() -> (w154:dbl)
        n81 = local read "ZPoints"() -> (w156:i32)
        n82 = call "Get position.vi"("Zaber"=w148, "error in"=w152) -> ("PositionRb"=w150:dbl, "error out"=w151:errorcluster)  [unwired: 13 in, 3 out]
        "ZEndPosition" <- w150
        n83 = local write "BtnSetZEndPosition"(FALSE ("BtnSetZEndPosition")) -> ()
        n84 = Decrement(x=w156) -> (x-1=w155:i32)
        n85 = Subtract(x=w150, y=w154) -> (x-y=w157:dbl)
        n86 = Divide(x=w157, y=w155) -> (x/y=w153:dbl)
        n87 = local write "ZStep"(w153) -> ()
      }
      event "ZPoints": Value Change {
        n88 = event-data() -> ("NewVal"=w161:i32)  [unwired: 1 in, 4 out]
        n89 = local read "ZEndPosition"() -> (w162:dbl)
        n90 = local read "ZStartPosition"() -> (w164:dbl)
        n91 = Decrement(x=w161) -> (x-1=w165:i32)
        n92 = Subtract(x=w162, y=w164) -> (x-y=w166:dbl)
        n93 = Divide(x=w166, y=w165) -> (x/y=w163:dbl)
        n94 = local write "ZStep"(w163) -> ()
      }
      event "btnStartFreqScanning": Value Change {
        w207 = 5
        n95 = event-data() -> ()  [unwired: 1 in, 5 out]
        n96 = local read "FrequencyPoints"() -> (w212:i32)
        n97 = for {
          N: w212 -> [_]
          tunnel: w216 -> [w255]
          tunnel: [w253] -> w176 mode=indexing
          tunnel: [w248] -> w211 mode=indexing
          shift-right: [w252] -> w213
          shift-left: w215 -> [w257]
          i -> [w262]
          w249 = T5 2 items=["X", "Y", "R", "Theta", "IN1", "IN2", "IN3", "IN4", "OUT1", "OUT2", "XNoise", "YNoise", "Phase", "SineOut", "DCLevel", "IntRefFreq", "ExtRefFreq"] ("DataChannel")
          n98 = local read "FrequencyStep"() -> (w263:dbl)
          n99 = local read "StartFrequency"() -> (w260:dbl)
          n100 = Multiply(x=w263, y=w262) -> (x*y=w261:dbl)
          n101 = Add(x=w260, y=w261) -> (x+y=w254:dbl)
          n102 = local write "Frequency"(w254) -> ()
          n103 = call "OutSineFreqSet.vi"("SR865 in"=w255, "Frequency"=w254, "error in"=w257) -> ("SR865 out"=w258:T1, "error out"=w259:errorcluster)  [unwired: 15 in]
          n104 = call "OutSineFreqGet.vi"("SR865 in"=w258, "error in"=w259) -> ("SR865 out"=w251:T1, "Frequency"=w253:dbl, "error out"=w256:errorcluster)  [unwired: 15 in]
          n105 = flat-sequence {
            tunnel: w256 -> [w264]
            tunnel: [w264] -> w250
            frame #0 {
              n106 = Wait (ms)(milliseconds to wait="SettingTime") -> ()  [unwired: 1 out]
            }
          }
          n107 = local write "FrequencyRb"(w253) -> ()
          n108 = call "DataChannelRead.vi"("SR865 in"=w251, "DataChannel"=w249, "error in"=w250) -> ("Signal"=w248:dbl, "error out"=w252:errorcluster)  [unwired: 14 in, 1 out]
          n109 = local write "Signal"(w248) -> ()
          "CurrentPoint" <- w262
        }
        n110 = local read "PltScanningFrequence"() -> (w210:cluster{dbl[], dbl[]}[])
        n111 = flat-sequence {
          tunnel: w213 -> [_]
          frame #0 {
            n112 = local write "btnStartFreqScanning"(FALSE ("btnStartStopScanningPosition")) -> ()
          }
        }
        n113 = local read "TipPlace"() -> (w168:u16)
        n114 = case shown="1" w168 {
          tunnel: w211 -> [w231 w241]
          tunnel: w210 -> [w233 w246]
          tunnel: w176 -> [w229 w244]
          tunnel: [w228 w243] -> w175
          tunnel: [w226 w236] -> w174
          tunnel: [w225 w238] -> w173
          tunnel: [w224 w240] -> w172
          tunnel: [w223 w237] -> w171
          tunnel: [w222 w235] -> w170
          frame 0, Default {
            n115 = Index Array(array=w233, index #1=0 ("index"), index #2=2 ("index"), index #3=3 ("index")) -> (element #1=w225:cluster{dbl[], dbl[]}, element #2=w224:cluster{dbl[], dbl[]}, element #3=w223:cluster{dbl[], dbl[]})
            n116 = Unbundle(w224) -> (w230:dbl[])  [unwired: 1 out]
            n117 = Subtract(x=w231, y=w230) -> (x-y=w228:dbl[])
            n118 = Bundle(w229, w231) -> (w226:cluster{dbl[], dbl[]})  [unwired: 1 in]
            n119 = Bundle(w229, w228) -> (w222:cluster{dbl[], dbl[]})  [unwired: 1 in]
          }
          frame 1 {
            n120 = Index Array(array=w246, index #1=0 ("index"), index #2=1 ("index"), index #3=2 ("index")) -> (element #1=w236:cluster{dbl[], dbl[]}, element #2=w238:cluster{dbl[], dbl[]}, element #3=w237:cluster{dbl[], dbl[]})
            n121 = Unbundle(w236) -> (w242:dbl[])  [unwired: 1 out]
            n122 = Subtract(x=w242, y=w241) -> (x-y=w243:dbl[])
            n123 = Bundle(w244, w241) -> (w240:cluster{dbl[], dbl[]})  [unwired: 1 in]
            n124 = Bundle(w244, w243) -> (w235:cluster{dbl[], dbl[]})  [unwired: 1 in]
          }
        }
        n125 = Build Array(w174, w173, w172, w171, w170) -> (→"PltScanningFrequence":cluster{dbl[], dbl[]}[])
        n126 = call <vilib>:"Peak Detector.vi"("peaks/valleys"=enum32{"Peaks", "Valleys"}."Peaks", "X"=w175) -> ("Amplitudes"=w199:dbl[], "Locations"=w188:dbl[], "# found"=w191:i32)  [unwired: 5 in, 2 out]
        n127 = call <vilib>:"Peak Detector.vi"("peaks/valleys"=enum32{"Peaks", "Valleys"}."Valleys", "X"=w175) -> ("Amplitudes"=w184:dbl[], "Locations"=w182:dbl[], "# found"=w192:i32)  [unwired: 5 in, 2 out]
        n128 = Negate(x=w184) -> (-x=w183:dbl[])
        n129 = Add(x=w191, y=w192) -> (x+y=w190:i32)
        n130 = Array Size(array=w188) -> (size(s)=w187:i32)
        n131 = Array Size(array=w182) -> (size(s)=w185:i32)
        n132 = Initialize Array(1, w187) -> (w181:i32[])
        n133 = Initialize Array(-1, w185) -> (w180:i32[])
        n134 = Build Cluster Array(w199, w188, w181) -> (w179:cluster{dbl, dbl, i32}[])
        n135 = Build Cluster Array(w183, w182, w180) -> (w178:cluster{dbl, dbl, i32}[])
        n136 = Insert Into Array(array=w179, new element=w178) -> (w177:cluster{dbl, dbl, i32}[])  [unwired: 1 in]
        n137 = Less Or Equal?(x=w207, y=w190) -> (x <= y?=w208:bool)
        n138 = Sort 1D Array(array=w177) -> (sorted array=w194:cluster{dbl, dbl, i32}[])
        n139 = Select(t=w207, s=w208, f=w190) -> (s? t:f=w198:i32)
        n140 = Reverse 1D Array(array=w194) -> (reversed array=w195:cluster{dbl, dbl, i32}[])
        n141 = for {
          N: w198 -> [_]
          tunnel: w195 -> [w221] mode=indexing
          tunnel: [w219] -> w196 mode=indexing
          tunnel: [w217] -> w197 mode=indexing
          n142 = Unbundle(w221) -> (w218:dbl, w219:dbl, w220:i32)
          n143 = Multiply(x=w218, y=w220) -> (x*y=w217:dbl)
        }
        n144 = local read "FrequencyStep"() -> (w206:dbl)
        n145 = local read "StartFrequency"() -> (w204:dbl)
        n146 = Multiply(x=w206, y=w196) -> (x*y=w205:dbl[])
        n147 = Add(x=w204, y=w205) -> (x+y=w203:dbl[])
        n148 = Build Array(w203, w197) -> (w202:dbl[][])
        n149 = Number To Fractional String(number=w202, precision (6)=i16 2) -> (F-format string=w200:string[][])  [unwired: 2 in]
        n150 = Transpose 2D Array(2D array=w200) -> (transposed array=→"TblBestFrequencyies":string[][])
      }
      event "btnStartPosScanning": Value Change {
        n151 = event-data() -> ()  [unwired: 1 in, 5 out]
        n152 = local read "ZPoints"() -> (w279:i32)
        n153 = for {
          N: w279 -> [_]
          tunnel: w269 -> [w281]
          shift-right: [w285] -> w267
          shift-left: w271 -> [w290]
          tunnel: [w288] -> w274 mode=indexing
          tunnel: [w282] -> w273 mode=indexing
          tunnel: w270 -> [w284]
          i -> [w291]
          w287 = T5 2 items=["X", "Y", "R", "Theta", "IN1", "IN2", "IN3", "IN4", "OUT1", "OUT2", "XNoise", "YNoise", "Phase", "SineOut", "DCLevel", "IntRefFreq", "ExtRefFreq"] ("DataChannel")
          n154 = local read "ZStep"() -> (w295:dbl)
          n155 = local read "ZStartPosition"() -> (w293:dbl)
          n156 = Increment(x=w291) -> (x+1=→"CurrentStep":i32)
          n157 = Multiply(x=w295, y=w291) -> (x*y=w294:dbl)
          n158 = Add(x=w293, y=w294) -> (x+y=w283:dbl)
          n159 = local write "ZPosition"(w283) -> ()
          n160 = call "Move absolute.vi"("Zaber"=w281, "Position, mm"=w283, "error in"=w290) -> ("Position, mm"=w288:dbl, "error out"=w289:errorcluster)  [unwired: 13 in, 2 out]
          n161 = flat-sequence {
            tunnel: [w297] -> w286
            tunnel: w289 -> [w297]
            frame #0 {
              n162 = local read "SettingTime"() -> (w296:u32)
              n163 = Wait (ms)(milliseconds to wait=w296) -> ()  [unwired: 1 out]
            }
          }
          n164 = local write "ZPositionRb"(w288) -> ()
          n165 = call "DataChannelRead.vi"("SR865 in"=w284, "DataChannel"=w287, "error in"=w286) -> ("Signal"=w282:dbl, "error out"=w285:errorcluster)  [unwired: 14 in, 1 out]
          n166 = local write "Signal"(w282) -> ()
        }
        n167 = local read "PltScanningPosition"() -> (w278:cluster{dbl[], dbl[]}[])
        n168 = Bundle(w274, w273) -> (w272:cluster{dbl[], dbl[]})  [unwired: 1 in]
        n169 = Index Array(array=w278, index=0) -> (element=w277:cluster{dbl[], dbl[]})
        n170 = Build Array(w272, w277) -> (→"PltScanningPosition":cluster{dbl[], dbl[]}[])
        n171 = flat-sequence {
          tunnel: w267 -> [_]
          frame #0 {
            n172 = local write "btnStartPosScanning"(FALSE ("btnStartPosScanning")) -> ()
          }
        }
      }
      event "btnCalculateAirLevel": Value Change {
        n173 = event-data() -> ()  [unwired: 1 in, 5 out]
        n174 = local read "PltScanningPosition"() -> (w301:cluster{dbl[], dbl[]}[])
        n175 = property on="PltScanningPosition" class="XYGraph (strict)"(error in=w303) -> (error out=w302:errorcluster, "CrsrList"=w321:T8)  [unwired: 1 in, 1 out]
        n176 = Index Array(array=w321, index #1=0 ("index"), index #2=1 ("index")) -> (element #1=w318:T9, element #2=w317:T9)
        n177 = Unbundle By Name(w318) -> ("Position.X"=w316:dbl)
        n178 = Unbundle By Name(w317) -> ("Position.X"=w313:dbl)
        n179 = Index Array(array=w301, index=0) -> (element=w300:cluster{dbl[], dbl[]})
        n180 = Unbundle(w300) -> (w315:dbl[], w314:dbl[])
        n181 = Search 1D Array(1D array=w315, element=w316) -> (index of element=w312:i32)  [unwired: 1 in]
        n182 = Search 1D Array(1D array=w315, element=w313) -> (index of element=w311:i32)  [unwired: 1 in]
        n183 = Max & Min(x=w312, y=w311) -> (max(x,y)=w310:i32, min(x,y)=w309:i32)
        n184 = Subtract(x=w310, y=w309) -> (x-y=w308:i32)
        n185 = Increment(x=w308) -> (x+1=w307:i32)
        n186 = Array Subset(array=w314, index=w309, length=w307) -> (w306:dbl[])
        n187 = call <vilib>:"Std Deviation and Variance.vi"("X"=w306) -> ("mean"=→"AirLevel":dbl, "standard deviation"=→"AirError":dbl)  [unwired: 1 in, 1 out]
      }
      event "btnCalculateSurfaceLevel": Value Change {
        n188 = event-data() -> ()  [unwired: 1 in, 5 out]
        n189 = local read "PltScanningPosition"() -> (w325:cluster{dbl[], dbl[]}[])
        n190 = property on="PltScanningPosition" class="XYGraph (strict)"(error in=w327) -> (error out=w326:errorcluster, "CrsrList"=w345:T8)  [unwired: 1 in, 1 out]
        n191 = Index Array(array=w345, index #1=0 ("index"), index #2=1 ("index")) -> (element #1=w342:T9, element #2=w341:T9)
        n192 = Index Array(array=w325, index=0) -> (element=w324:cluster{dbl[], dbl[]})
        n193 = Unbundle By Name(w342) -> ("Position.X"=w340:dbl)
        n194 = Unbundle By Name(w341) -> ("Position.X"=w337:dbl)
        n195 = Unbundle(w324) -> (w339:dbl[], w338:dbl[])
        n196 = Search 1D Array(1D array=w339, element=w340) -> (index of element=w336:i32)  [unwired: 1 in]
        n197 = Search 1D Array(1D array=w339, element=w337) -> (index of element=w335:i32)  [unwired: 1 in]
        n198 = Max & Min(x=w336, y=w335) -> (max(x,y)=w334:i32, min(x,y)=w333:i32)
        n199 = Subtract(x=w334, y=w333) -> (x-y=w332:i32)
        n200 = Increment(x=w332) -> (x+1=w331:i32)
        n201 = Array Subset(array=w338, index=w333, length=w331) -> (w330:dbl[])
        n202 = call <vilib>:"Std Deviation and Variance.vi"("X"=w330) -> ("mean"=→"SurfaceLevel":dbl, "standard deviation"=→"SurfaceError":dbl)  [unwired: 1 in, 1 out]
      }
      event "btnCalculateSlope": Value Change {
        w355 = T10 0 items=["Least Square", "Least Absolute Residual", "Bisquare"] ("method")
        n203 = event-data() -> ()  [unwired: 1 in, 5 out]
        n204 = local read "PltScanningPosition"() -> (w349:cluster{dbl[], dbl[]}[])
        n205 = property on="PltScanningPosition" class="XYGraph (strict)"(error in=w351) -> (error out=w350:errorcluster, "CrsrList"=w372:T8)  [unwired: 1 in, 1 out]
        n206 = Index Array(array=w372, index #1=0 ("index"), index #2=1 ("index")) -> (element #1=w369:T9, element #2=w368:T9)
        n207 = Index Array(array=w349, index=0) -> (element=w348:cluster{dbl[], dbl[]})
        n208 = Unbundle By Name(w369) -> ("Position.X"=w367:dbl)
        n209 = Unbundle By Name(w368) -> ("Position.X"=w365:dbl)
        n210 = Unbundle(w348) -> (w360:dbl[], w366:dbl[])
        n211 = Search 1D Array(1D array=w360, element=w367) -> (index of element=w364:i32)  [unwired: 1 in]
        n212 = Search 1D Array(1D array=w360, element=w365) -> (index of element=w363:i32)  [unwired: 1 in]
        n213 = Max & Min(x=w364, y=w363) -> (max(x,y)=w362:i32, min(x,y)=w358:i32)
        n214 = Subtract(x=w362, y=w358) -> (x-y=w361:i32)
        n215 = Increment(x=w361) -> (x+1=w359:i32)
        n216 = Array Subset(array=w360, index=w358, length=w359) -> (w356:dbl[])
        n217 = Array Subset(array=w366, index=w358, length=w359) -> (w357:dbl[])
        n218 = call <vilib>:"Linear Fit.vi"("Y"=w357, "X"=w356, "method"=w355) -> ("slope"=w353:dbl, "residue"=→"SlopeError":dbl)  [unwired: 8 in, 3 out]
        n219 = Reciprocal(x=w353) -> (1/x=→"Slope":dbl)
      }
    }
  }
  "error out" <- w6
  "PhaseRb" <- "Phase"
